vi "Read View Channel info.vi"(8 "error in":errorcluster, 11 "channel in":refnum<class "channel node.lvclass">) -> (0 "error out":errorcluster, 2 "channel info":T1, 3 "channel out":refnum<class "channel node.lvclass">)   [LabVIEW 2013, in "channel node.lvclass"]
uses:
  channel node.lvclass
  ChannelDisplayInfo.ctl
  channel node.lvclass/channel node.ctl
  channel configuration/channel configuration.lvclass/channel configuration.ctl
  channel configuration/Read IO.vi
  channel configuration/Read sensor ID.vi
  channel configuration/Read channel name.vi
  channel configuration/Read description.vi
  channel configuration/channel configuration.lvclass
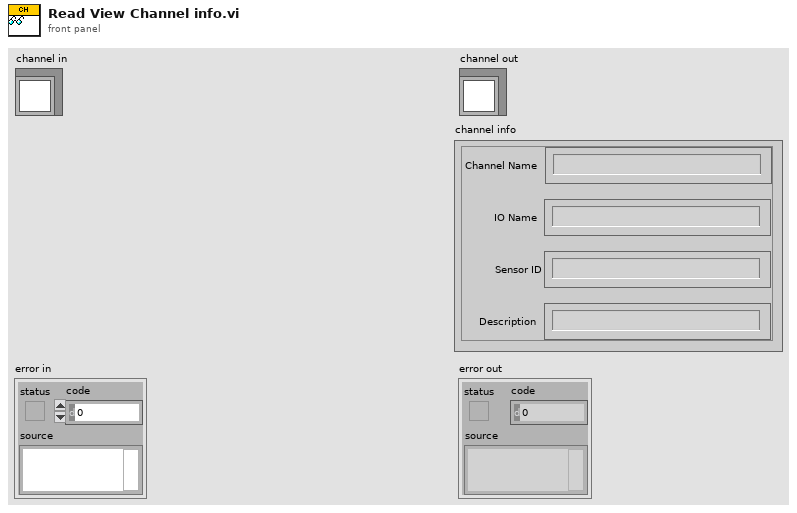
[diagram p1: front panel]
types:
  T1 = typedef "channel node.lvclass/ChannelDisplayInfo.ctl" = cluster{"IO Name":string, "Sensor ID":string, "Channel Name":string, "Description ":string}
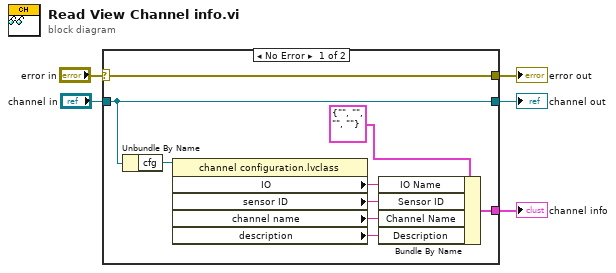
[diagram p0: block diagram]
diagram:
  n1 = case shown="No Error" "error in" {
    selector: "error in" -> [w14 w15]
    tunnel: [w14 w15] -> w4
    tunnel: [w13 w16] -> w2
    tunnel: "channel in" -> [w13 w16]
    tunnel: [w12 _] -> w1
    frame No Error {
      n2 = Unbundle By Name(w13) -> ("cfg"=w10:refnum<class "channel configuration.lvclass">)
      n3 = property class="channel configuration.lvclass"(reference=w10) -> ("IO "=w9:string, "sensor ID"=w8:string, "channel name"=w7:string, "description"=w6:string)  [unwired: 1 in, 2 out]
      n4 = Bundle By Name(cluster=T1 {"IO Name"="", "Sensor ID"="", "Channel Name"="", "Description "=""} ("channel info"), "IO Name"=w9, "Sensor ID"=w8, "Channel Name"=w7, "Description"=w6) -> (w12:T1)
    }
    frame Error {
    }
  }
  "error out" <- w4
  "channel out" <- w2
  "channel info" <- w1
